vi "Generate Calibrated Chirp Waveform.vi"(0 "TSM context In":T1, 1 "dB SPL":dbl, 5 "Start Freq (Hz)":dbl, 7 "Stop Freq (Hz)":dbl, 9 "Samples":i32, 11 "error in (no error)":errorcluster, 12 "Sampling Rate (Hz)":dbl) -> (4 "TSM context Out":T1, 6 "Per Site Waveform":waveform(dbl)[](array[waveform]), 15 "error out":errorcluster)   [LabVIEW 2020]
doc: "VI generates a calibrated Chirp Waveform from start to stop frequency at the given dB SPL"
uses:
  <vilib>/NI_TestStand_SemiconductorModule/NI_TestStand_Semiconductor_Module.lvlibp/PinMap/General/SemiconductorModuleContext.ctl
  <vilib>/Analysis/1siggen.llb/Ramp Pattern by Samples.vi
  <vilib>/Analysis/NI_AALBase.lvlib
  <vilib>/NI_TestStand_SemiconductorModule/NI_TestStand_Semiconductor_Module.lvlibp
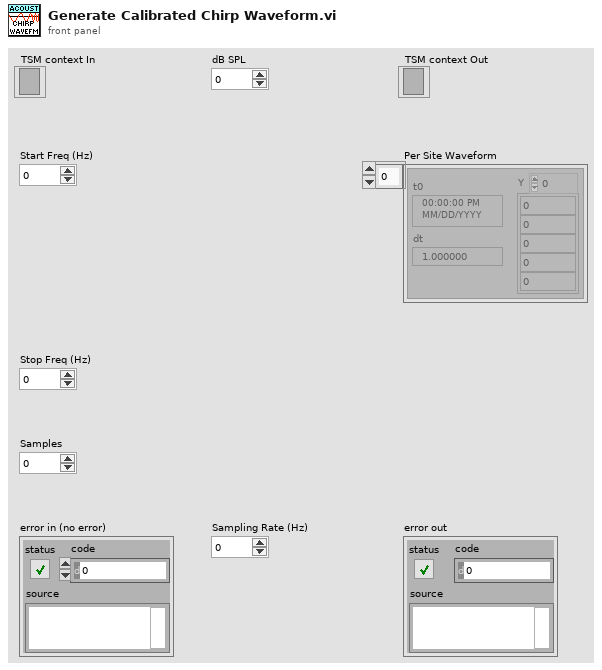
[diagram p1: front panel]
types:
  T1 = typedef "NI_TestStand_Semiconductor_Module.lvlibp/SemiconductorModuleContext.ctl" = refnum<k7>
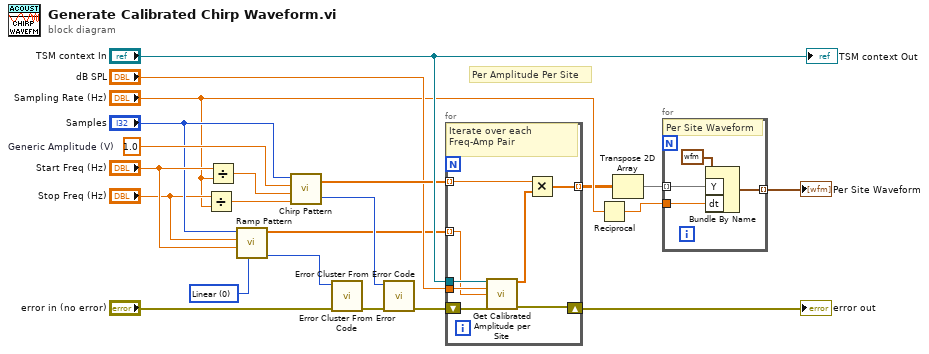
[diagram p0: block diagram]
diagram:
  w14 = u16 0 items=["Linear", "Logarithmic"] ("type")
  w15 = 1.0  # Generic Amplitude (V)
  # "Per Amplitude Per Site"
  n1 = Divide(x="Stop Freq (Hz)", y="Sampling Rate (Hz)") -> (x/y=w3:dbl)
  n2 = Divide(x="Start Freq (Hz)", y="Sampling Rate (Hz)") -> (x/y=w6:dbl)
  n3 = call-poly <vilib>:"Ramp Pattern.vi"("type"=w14, "start"="Start Freq (Hz)", "end"="Stop Freq (Hz)", "samples"="Samples") -> ("error"=w8:i32, "Ramp Pattern"=w11:dbl[])  [unwired: 6 in]
  n4 = call <vilib>:"Chirp Pattern.vi"("f2"=w3, "f1"=w6, "amplitude"=w15, "samples"="Samples") -> ("error"=w17:i32, "Chirp Pattern"=w19:dbl[])
  n5 = call <vilib>:"Error Cluster From Error Code.vi"("error in (no error)"="error in (no error)", "error code (0)"=w8) -> ("error out"=w9:errorcluster)  [unwired: 7 in]
  n6 = call <vilib>:"Error Cluster From Error Code.vi"("error in (no error)"=w9, "error code (0)"=w17) -> ("error out"=w18:errorcluster)  [unwired: 7 in]
  n7 = for {
    tunnel: "dB SPL" -> [w30]
    tunnel: "TSM context In" -> [w29]
    shift-right: [w27] -> w21
    shift-left: w18 -> [w28]
    tunnel: w19 -> [w26] mode=indexing
    tunnel: [w24] -> w2 mode=indexing
    tunnel: w11 -> [w23] mode=indexing
    # "Iterate over each Freq-Amp Pair"
    n8 = call "Get Calibrated Amplitude per Site.vi"("TSM context"=w29, "dB SPL"=w30, "Frequency (Hz)"=w23, "error in (no error)"=w28) -> ("Per Site Amplitude (V)"=w25:dbl[], "error out"=w27:errorcluster)  [unwired: 9 in, 1 out]
    n9 = Multiply(x=w26, y=w25) -> (x*y=w24:dbl[])
  }
  "error out" <- w21
  n10 = Reciprocal(x="Sampling Rate (Hz)") -> (1/x=w22:dbl)
  n11 = Transpose 2D Array(2D array=w2) -> (transposed array=w1:dbl[][])
  n12 = for {
    tunnel: w1 -> [w34] mode=indexing
    tunnel: [w32] -> w7 mode=indexing
    tunnel: w22 -> [w31]
    # "Per Site Waveform"
    n13 = Bundle By Name(cluster=waveform(dbl) {"t0"=timestamp(0 s since 1904-01-01), "dt"=1.0, "Y"=[]} ("waveform"), "Y"=w34, "dt"=w31) -> (w32:waveform(dbl))
  }
  "Per Site Waveform" <- w7
  "TSM context Out" <- "TSM context In"
